vi "EXCOM-COM-WRITE.vi"(0 "VRN IN":refnum<visa-resource-name>="-1", 2 "Commande #":i32=-1, 7 "Args":dbl[](array[numeric]) format="%.2f", 11 "Error IN":errorcluster) -> (4 "VRN OUT":refnum<visa-resource-name>="-1", 8 "OK Done":bool, 15 "Error OUT":errorcluster)   [LabVIEW 2011]
panel:
  out "Cmd String":string
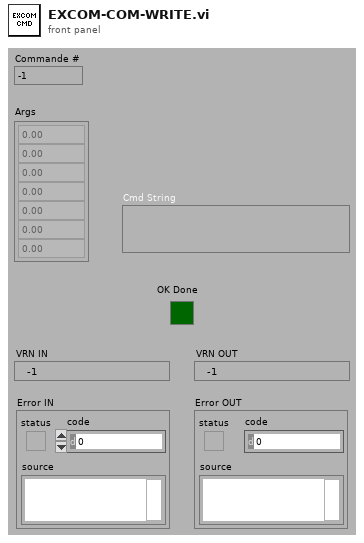
[diagram p1: front panel]
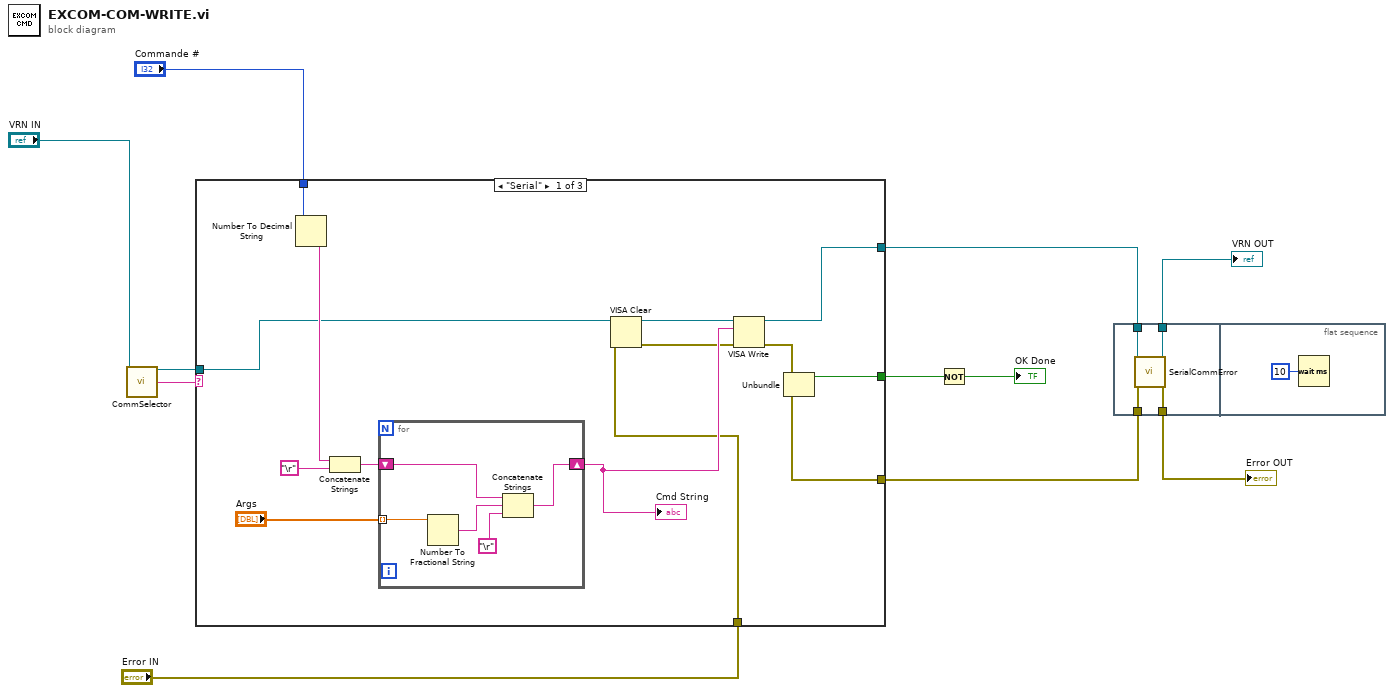
[diagram p0: block diagram]
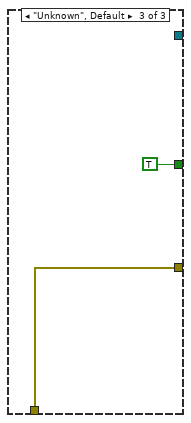
[diagram p3: hidden frame]
diagram:
  n1 = call "CommSelector.vi"("VISA resource name"="VRN IN") -> ("VISA resource name"=w2:refnum<visa-resource-name>, "CommType"=w3:string)  [unwired: 13 in]
  n2 = case shown="\"Serial\"" w3 {
    tunnel: [w24 _ TRUE ("status")] -> w10
    tunnel: [w22 _ w31] -> w7
    tunnel: "Error IN" -> [w16 _ w31]
    tunnel: [w17 _ w30] -> w8
    tunnel: w2 -> [w13 _ _]
    tunnel: "Commande #" -> [w12 _ _]
    frame "Serial" {
      n3 = Number To Decimal String(number=w12) -> (decimal integer string=w19:string)  [unwired: 1 in]
      n4 = Concatenate Strings(w19, "\r") -> (w20:string)
      n5 = for {
        shift-right: [w27] -> w23
        shift-left: w20 -> [w29]
        tunnel: "Args" -> [w26] mode=indexing
        n6 = Number To Fractional String(number=w26) -> (F-format string=w25:string)  [unwired: 3 in]
        n7 = Concatenate Strings(w29, w25, "\r") -> (w27:string)
      }
      "Cmd String" <- w23
      n8 = VISA Clear(VISA resource name=w13, error in (no error)=w16) -> (VISA resource name out=w15:refnum<visa-resource-name>, error out=w14:errorcluster)
      n9 = VISA Write(VISA resource name=w15, write buffer=w23, error in (no error)=w14) -> (VISA resource name out=w17:refnum<visa-resource-name>, error out=w22:errorcluster)  [unwired: 1 out]
      n10 = Unbundle(w22) -> ("status"=w24:bool)  [unwired: 2 out]
    }
    frame "TCP/IP" {
    }
    frame "Unknown", Default {
    }
  }
  n11 = Not(x=w10) -> (.not. x?=→"OK Done":bool)
  n12 = flat-sequence {
    tunnel: w8 -> [w36]
    tunnel: w7 -> [w35]
    tunnel: [w34] -> w6
    tunnel: [w33] -> w5
    frame #0 {
      n13 = call "SerialCommError.vi"("VISA IN"=w36, "error IN"=w35) -> ("VISA OUT"=w34:refnum<visa-resource-name>, "error OUT"=w33:errorcluster)  [unwired: 11 in, 1 out]
    }
    frame #1 {
      n14 = Wait (ms)(milliseconds to wait=u32 10) -> ()  [unwired: 1 out]
    }
  }
  "VRN OUT" <- w6
  "Error OUT" <- w5
